vi "RD_Program_result.vi"(6 "Match_Score":dbl, 7 "Offset array":dbl[](array[numeric]), 8 "lower limit":dbl=2.1 format="%#_13g", 9 "upper limit":dbl, 10 "name":string="123.txt", 11 "base path":path) -> (0 "data":T1, 1 "結果":bool, 2 "path":path, 3 "數據結果":string)   [LabVIEW 2019]
uses:
  <vilib>/regexp/Match Regular Expression.xnode
panel:
  out "Numeric":i32
  out "超過範圍NG":bool[](array[boolean])
  out "text":string
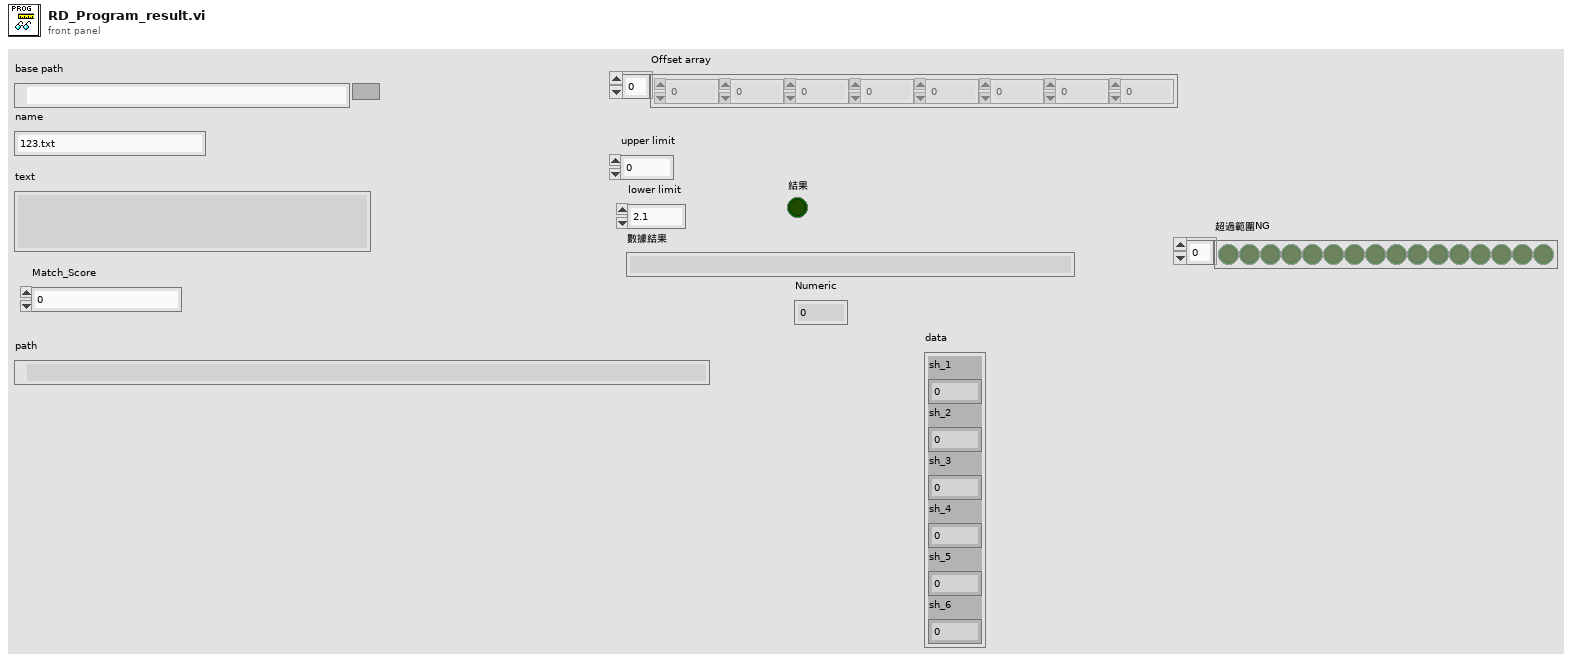
[diagram p1: front panel]
types:
  T1 = cluster{"sh_1":dbl, "sh_2":dbl, "sh_3":dbl, "sh_4":dbl, "sh_5":dbl, "sh_6":dbl}
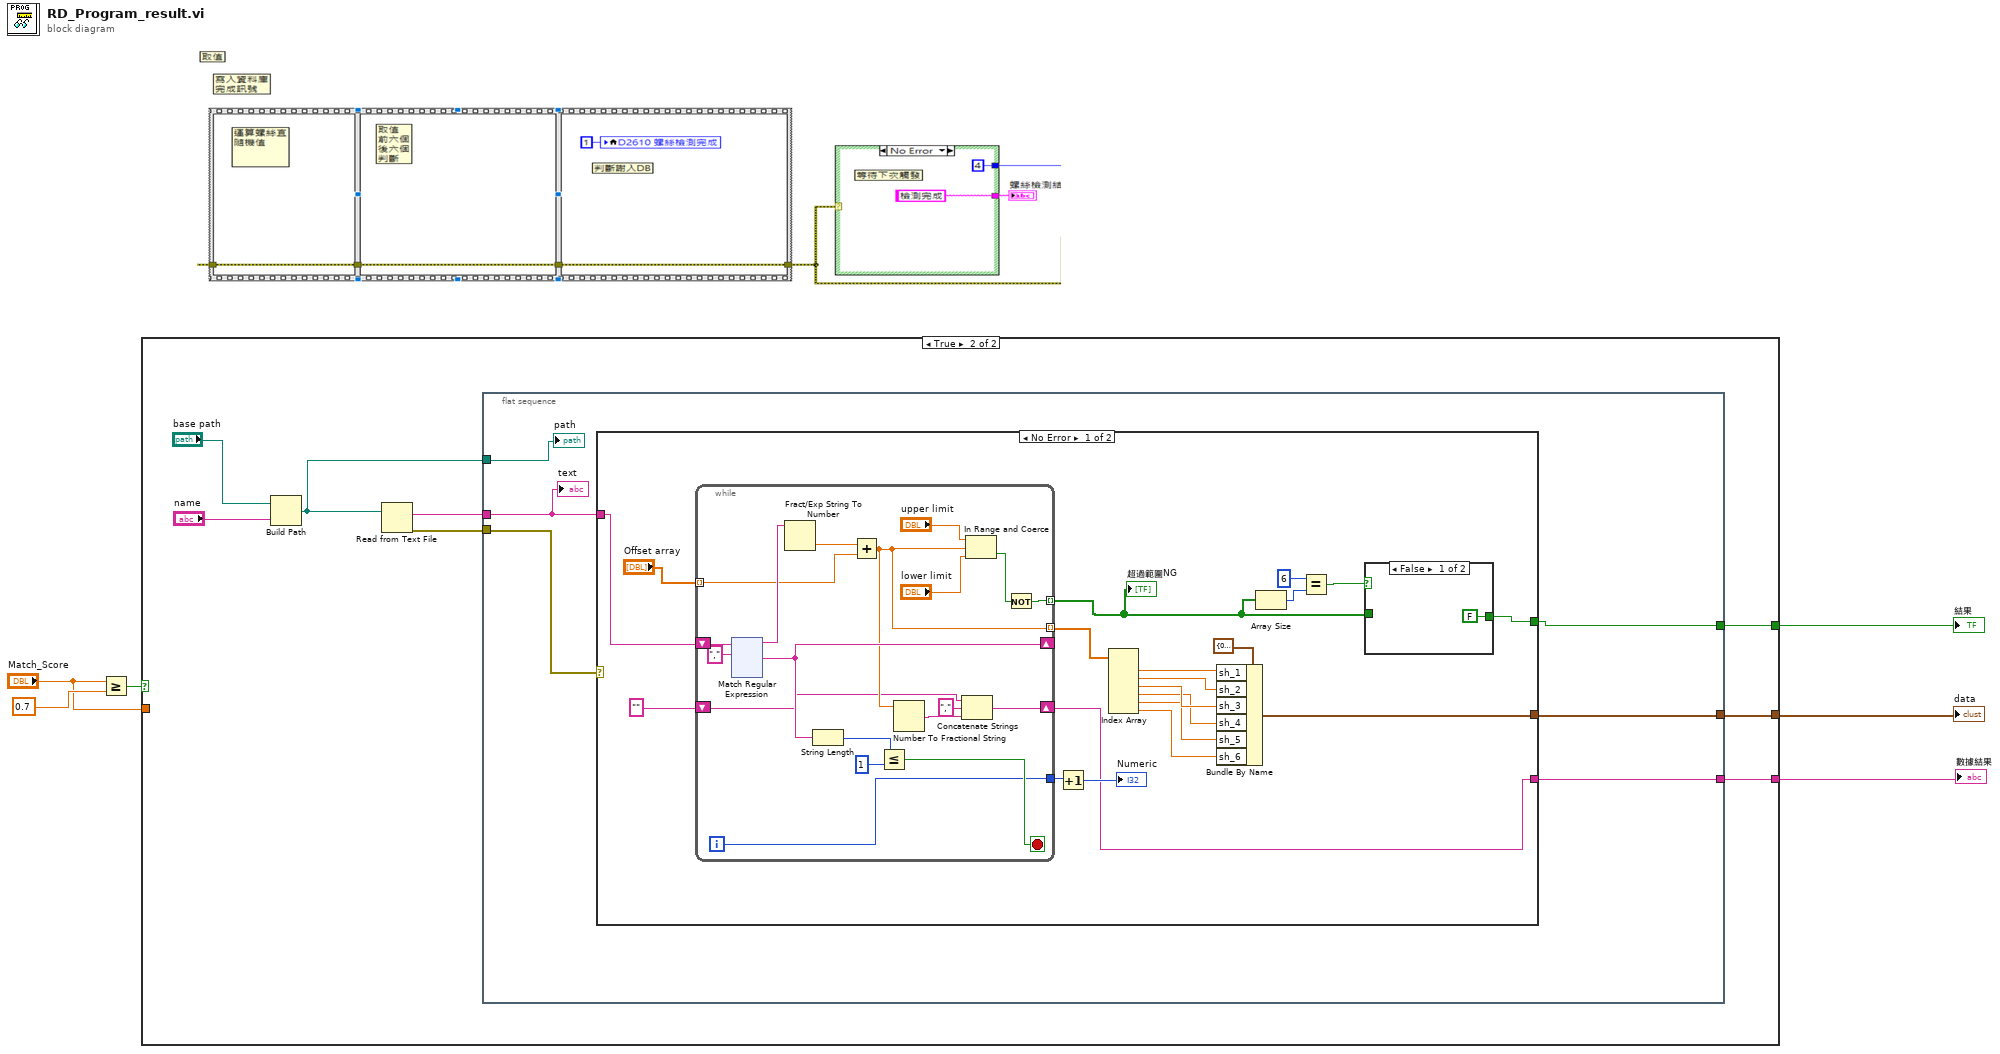
[diagram p0: block diagram]
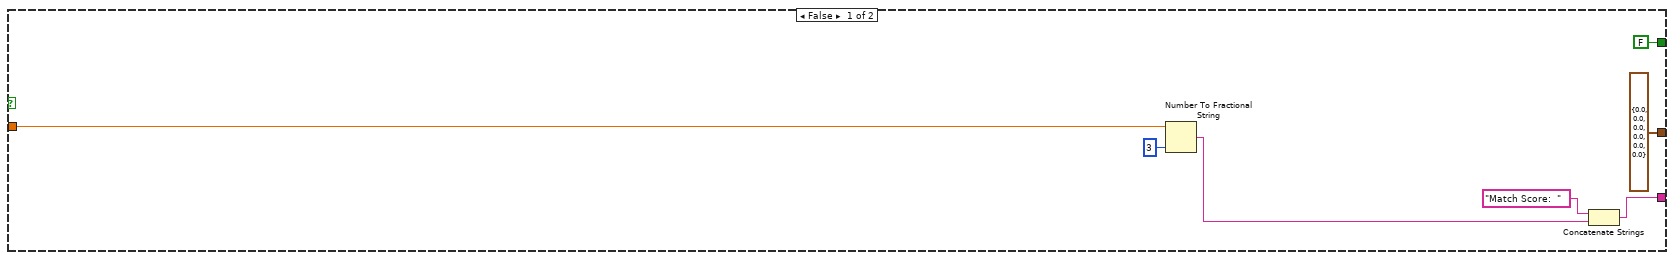
[diagram p2: hidden frame]
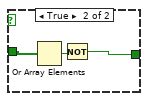
[diagram p3: hidden frame]
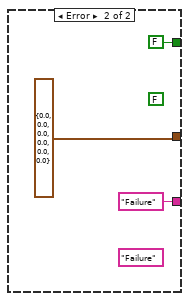
[diagram p4: hidden frame]
diagram:
  n1 = Greater Or Equal?(x="Match_Score", y=0.7) -> (x >= y?=w2:bool)
  n2 = case shown="True" w2 {
    tunnel: [w7 w16] -> w6
    tunnel: [T1 {"sh_1"=0.0, "sh_2"=0.0, "sh_3"=0.0, "sh_4"=0.0, "sh_5"=0.0, "sh_6"=0.0} w15] -> w5
    tunnel: [FALSE w14] -> w4
    tunnel: "Match_Score" -> [w11 _]
    frame False {
      n3 = Number To Fractional String(number=w11, precision (6)=i16 3) -> (F-format string=w8:string)  [unwired: 2 in]
      n4 = Concatenate Strings("Match Score:  ", w8) -> (w7:string)
    }
    frame True {
      n5 = Build Path(base path="base path", name or relative path="name") -> (appended path=w17:path)
      n6 = Read from Text File(file (use dialog)=w17) -> (text=w20:string, error out=w21:errorcluster)  [unwired: 3 in, 2 out]
      n7 = flat-sequence {
        tunnel: w21 -> [w26]
        tunnel: w20 -> [w27]
        tunnel: w17 -> [w25]
        tunnel: [w24] -> w16
        tunnel: [w23] -> w15
        tunnel: [w22] -> w14
        frame #0 {
          n8 = case shown="No Error" w26 {
            tunnel: [w29 "Failure"] -> w24
            tunnel: w27 -> [w43 _]
            tunnel: [w47 FALSE] -> w22
            tunnel: [w31 T1 {"sh_1"=0.0, "sh_2"=0.0, "sh_3"=0.0, "sh_4"=0.0, "sh_5"=0.0, "sh_6"=0.0}] -> w23
            frame No Error {
              n9 = while {
                shift-right: [w58] -> _
                shift-left: w43 -> [w69]
                tunnel: [w64] -> w42 mode=indexing
                tunnel: [w60] -> w41
                tunnel: [w57] -> w39 mode=indexing
                shift-right: [w53] -> w29
                shift-left: "" -> [w54]
                tunnel: "Offset array" -> [w52] mode=indexing
                i -> [w60]
                stop <- w61 stop-if-true
                n10 = xnode "Match Regular Expression"("input string"=w69, "regular expression"=",") -> ("before match"=w68:string, "after match"=w58:string)  [unwired: 4 in, 3 out]
                n11 = Fract/Exp String To Number(string=w68) -> (number=w59:dbl)  [unwired: 3 in, 1 out]
                n12 = String Length(string=w58) -> (length=w63:i32)
                n13 = Add(x=w59, y=w52) -> (x+y=w57:dbl)
                n14 = Less Or Equal?(x=w63, y=1) -> (x <= y?=w61:bool)
                n15 = Number To Fractional String(number=w57) -> (F-format string=w55:string)  [unwired: 3 in]
                n16 = Concatenate Strings(w54, "," ("string"), w55) -> (w53:string)
                n17 = In Range and Coerce(upper limit="upper limit", x=w57, lower limit="lower limit") -> (In Range?=w65:bool)  [unwired: 1 out]
                n18 = Not(x=w65) -> (.not. x?=w64:bool)
              }
              "超過範圍NG" <- w42
              n19 = Increment(x=w41) -> (x+1=→"Numeric":i32)
              n20 = Index Array(array=w39) -> (element #1=w37:dbl, element #2=w36:dbl, element #3=w35:dbl, element #4=w34:dbl, element #5=w33:dbl, element #6=w32:dbl)  [unwired: 6 in]
              n21 = Bundle By Name(cluster=T1 {"sh_1"=0.0, "sh_2"=0.0, "sh_3"=0.0, "sh_4"=0.0, "sh_5"=0.0, "sh_6"=0.0}, "sh_1"=w37, "sh_2"=w36, "sh_3"=w35, "sh_4"=w34, "sh_5"=w33, "sh_6"=w32) -> (w31:T1)
              n22 = Array Size(array=w42) -> (size(s)=w45:i32)
              n23 = Equal?(x=6, y=w45) -> (x = y?=w46:bool)
              n24 = case shown="False" w46 {
                tunnel: w42 -> [_ w51]
                tunnel: [FALSE w49] -> w47
                frame False {
                }
                frame True {
                  n25 = Or Array Elements(Boolean array=w51) -> (logical OR=w50:bool)
                  n26 = Not(x=w50) -> (.not. x?=w49:bool)
                }
              }
            }
            frame Error {
              (unwired) FALSE
              (unwired) "Failure"
            }
          }
          "text" <- w27
          "path" <- w25
        }
      }
    }
  }
  "數據結果" <- w6
  "data" <- w5
  "結果" <- w4
